vi "Write OCP Delay.vi"(8 "error in":errorcluster, 10 "Delay":dbl, 11 "Electronic Load in":refnum<class "Electronic Load.lvclass">) -> (0 "error out":errorcluster, 3 "Electronic Load out":refnum<class "Electronic Load.lvclass">)   [LabVIEW 2019, in "Electronic Load.lvlib" / "Electronic Load.lvclass"]
uses:
  Library/Electronic Load.lvclass
  C:/Users/Public/Documents/Development/builds/Instruments/Instruments.lvlibp/Library/Instruments.lvclass
  Library/Electronic Load.lvclass/Electronic Load.ctl
  builds/Instruments/Instruments.lvlibp/Private/Polymorphic/Integers/Event from DBL.vi
  builds/Instruments/Instruments.lvlibp/Accessors/Command with Logging.vi
  builds/Instruments/Instruments.lvlibp/Library/Instruments.lvclass
  builds/Instruments/Instruments.lvlibp
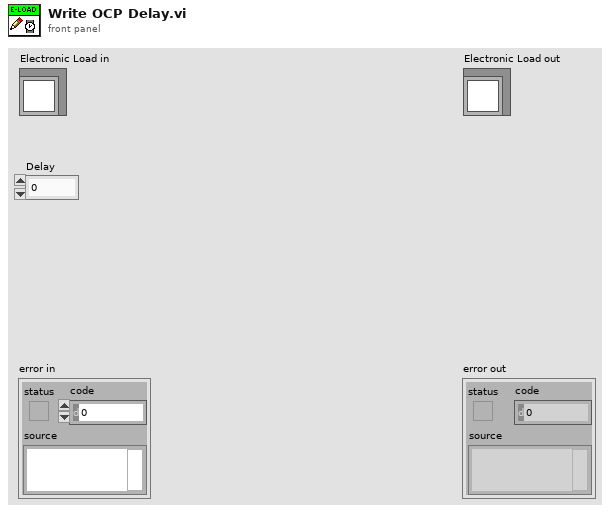
[diagram p1: front panel]
types:
  T1 = typedef "Electronic Load.lvlib/Electronic Load.lvclass/OCP Settings.ctl" = cluster{"OCP_Enabled":bool, "OCP Level":dbl, "OCP Delay":dbl}
  T2 = cluster{"Timestamp":timestamp, "Description":string, "Data":string}
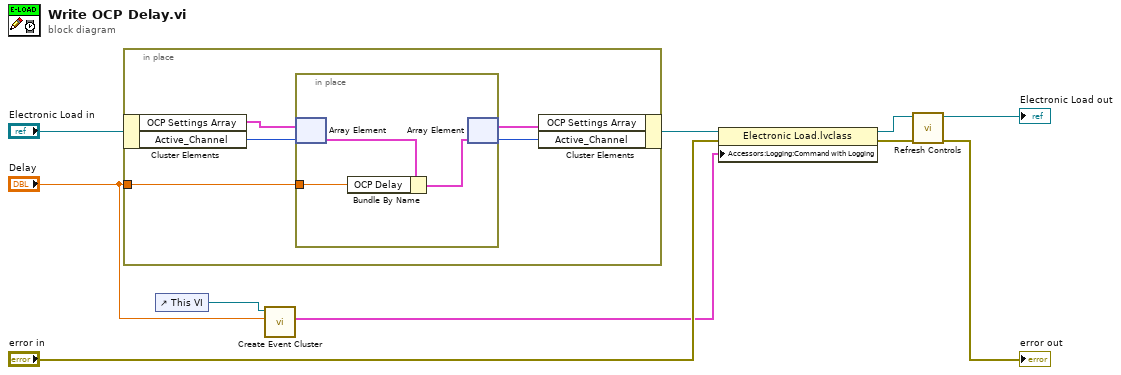
[diagram p0: block diagram]
diagram:
  n1 = in-place {
    in-place-border: "Delay" -> [w11]
    n2 = in-place-cluster #1("Electronic Load in") -> ("OCP Settings Array"=w15:T1[], "Active_Channel"=w14:u32)
    n3 = in-place {
      in-place-border: w11 -> [w16]
      n4 = in-place-array #2(w15, w14) -> (w18:T1)
      n5 = Bundle By Name(cluster=w18, "OCP Delay"=w16) -> (w17:T1)
      n6 = in-place-array #2(w17) -> (w13:T1[], w12:i32)
    }
    n7 = in-place-cluster #1("OCP Settings Array"=w13, "Active_Channel"=w12) -> (w7:refnum<class "Electronic Load.lvclass">)
  }
  n8 = control-ref of="This VI"() -> (w9:refnum<vi>)
  n9 = call-poly "Create Event Cluster.vi"("Value"="Delay", "VI Refnum"=w9) -> ("Event Data"=w5:T2)  [unwired: 9 in]
  n10 = property class="Electronic Load.lvclass"(reference=w7, error in="error in", "Accessors:Logging:Command with Logging"=w5) -> (reference out=w4:refnum<class "Electronic Load.lvclass">, error out=w3:errorcluster)
  n11 = call "Refresh Controls.vi"("error in"=w3, "Electronic Load in"=w4) -> ("error out"=→"error out":errorcluster, "Electronic Load out"=→"Electronic Load out":refnum<class "Electronic Load.lvclass">)  [unwired: 8 in]
